vi "PS-RA01B FPGA Testbench.vi"() -> ()   [LabVIEW 2011]
uses:
  <vilib>/rvi/eio/common/nirviEmuTemplateMethod_errors.vi
  <vilib>/rvi/Memory/Memory_Emulation/niFpgaMemoryEmulationValidateCache.vi
  <vilib>/rvi/DataTransferAndStorage/Container/Common/niFpgaContainerGetUniqueNameForEmu.vi
  <vilib>/rvi/Memory/Memory_Emulation/nirvimemoryEmulationManagerCache_InsertValue.vi
  <vilib>/Utility/error.llb/Clear Errors.vi
  <vilib>/rvi/Memory/Memory_Emulation/nirvimemoryEmulationManagerCache_GetValue.vi
  <vilib>/rvi/Memory/Memory_Emulation/nirvimemoryEmulationManagerCache_SetValue.vi
  <vilib>/eio/EIONode/EIONode.xnode
  <vilib>/eio/EIOMethodNode/EIOMethodNode.xnode
  <vilib>/rvi/DataTransferAndStorage/Container/XNode/niFpgaContainer.xnode
  <vilib>/rvi/Memory/Memory_Emulation/nirvimemoryEmulation.vi
panel:
  out "ADDR":u8
  out "Mod6/AO1":fxp<+/-,20,5> format="%.17g"
  out "Mod2/AO3":fxp<+/-,20,5> format="%.17g"
  out "Mod2/AO2":fxp<+/-,20,5> format="%.17g"
  out "Mod2/AO1":fxp<+/-,20,5> format="%.17g"
  out "Mod2/AO0":fxp<+/-,20,5> format="%.17g"
  out "Mod6/AO3":fxp<+/-,20,5> format="%.17g"
  out "Mod6/AO2":fxp<+/-,20,5> format="%.17g"
  out "Mod6/AO0":fxp<+/-,20,5> format="%.17g"
  out "Timestamp":u32 caption="Tick Count(Ticks)"
  out "Mod5/AI0":fxp<+/-,20,5> format="%.17g"
  out "Mod5/AI2":fxp<+/-,20,5> format="%.17g"
  out "Mod5/AI3":fxp<+/-,20,5> format="%.17g"
  out "Mod1/AI0":fxp<+/-,20,5> format="%.17g"
  out "Mod1/AI1":fxp<+/-,20,5> format="%.17g"
  out "Mod1/AI2":fxp<+/-,20,5> format="%.17g"
  out "Mod1/AI3":fxp<+/-,20,5> format="%.17g"
  out "Mod5/AI1":fxp<+/-,20,5> format="%.17g"
  out "period":u32
  out "delay":u32
  out "dperiod":u32
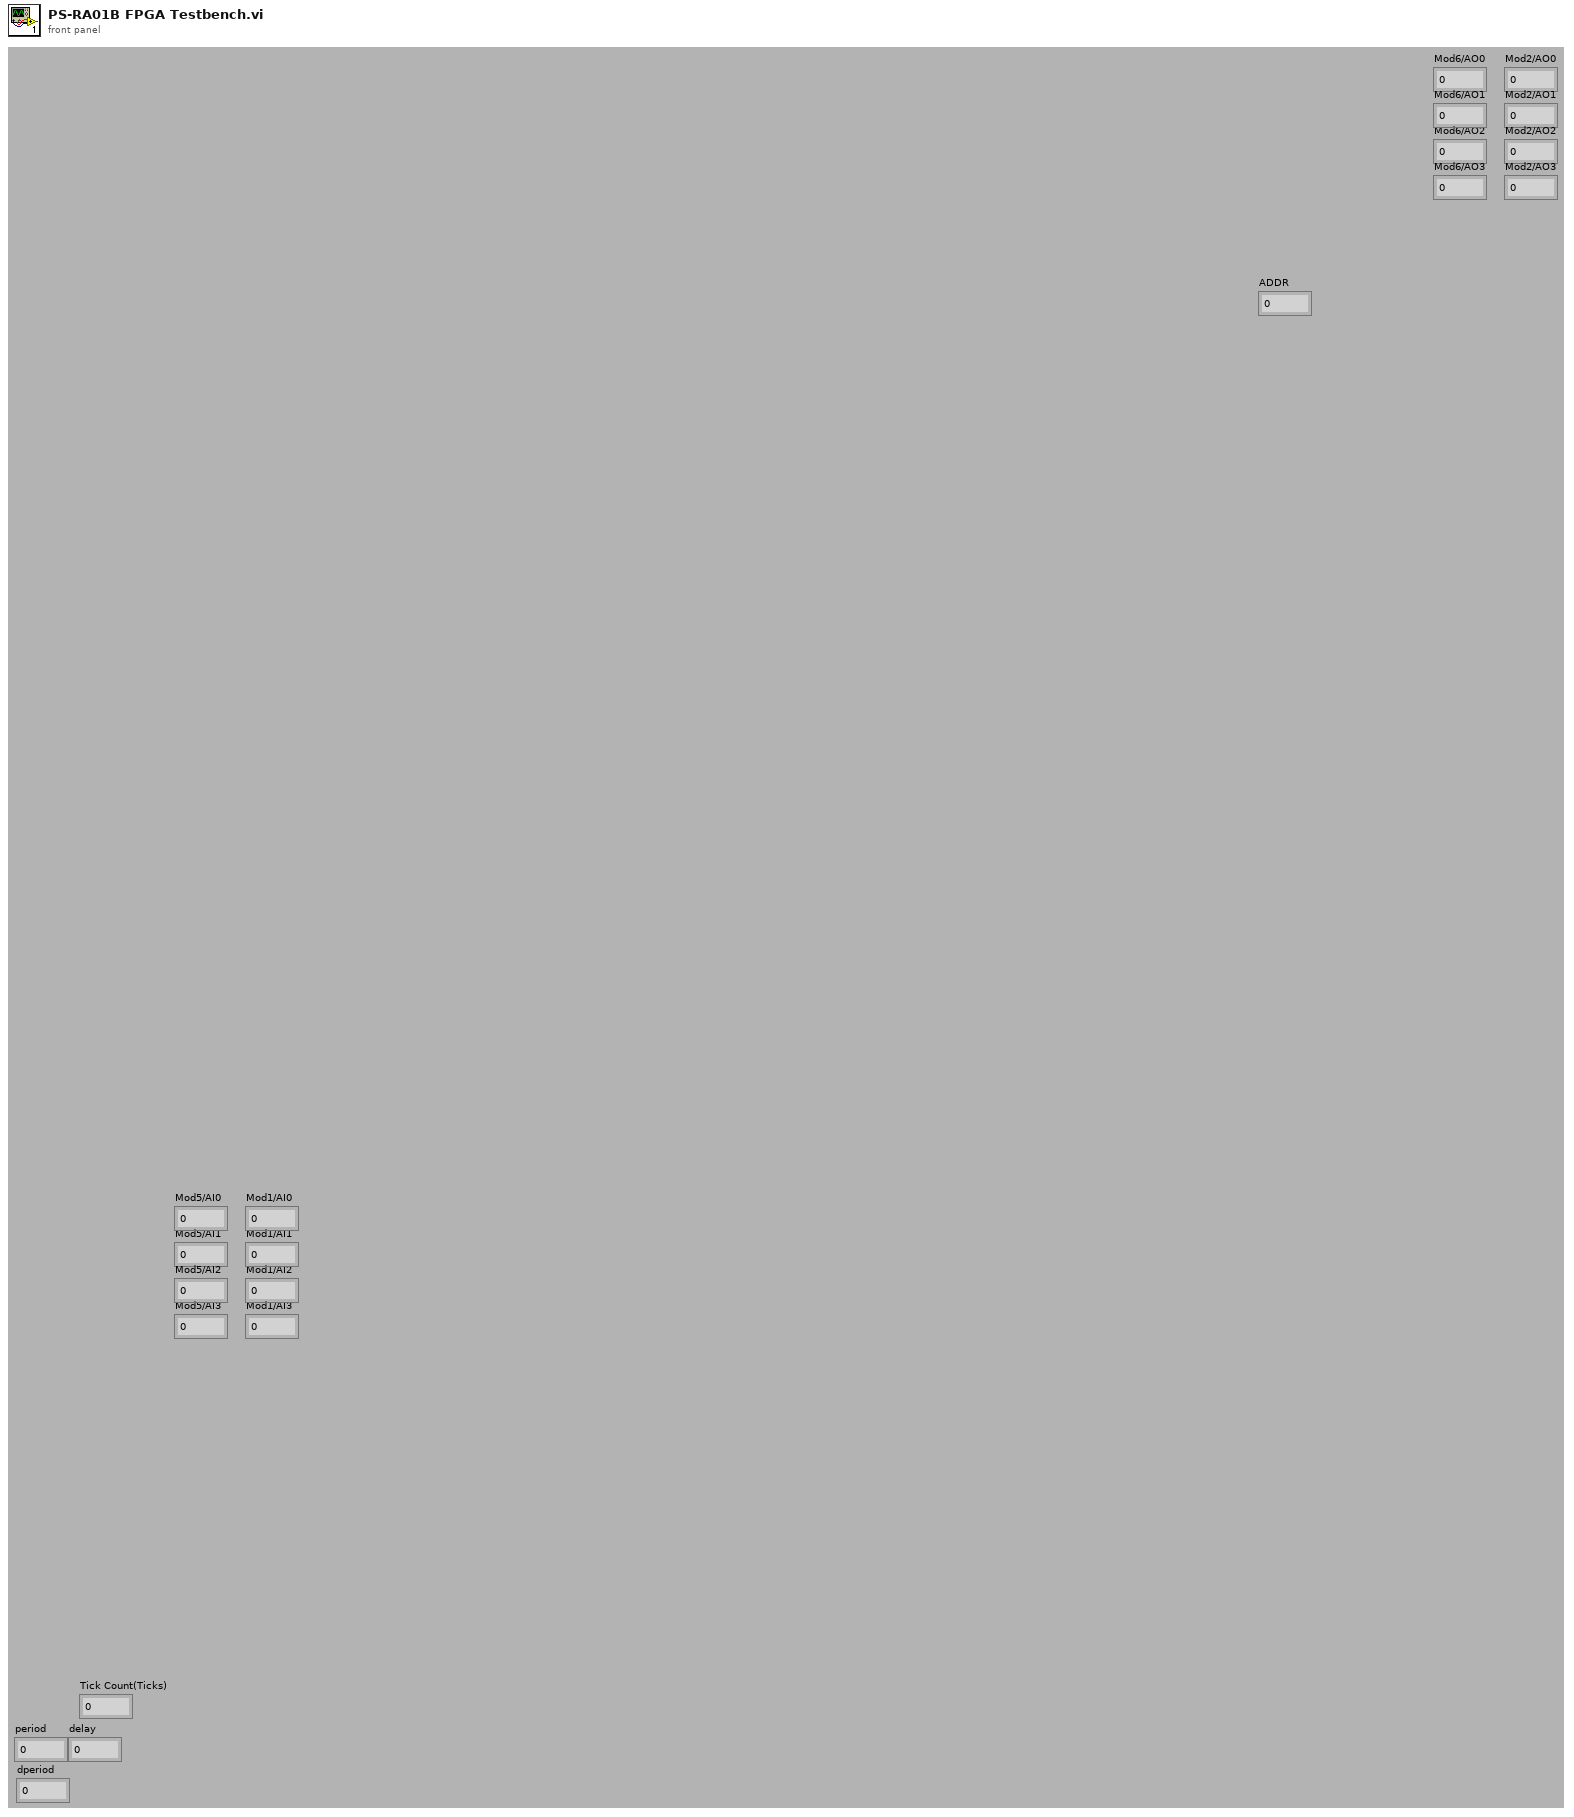
[diagram p1: front panel]
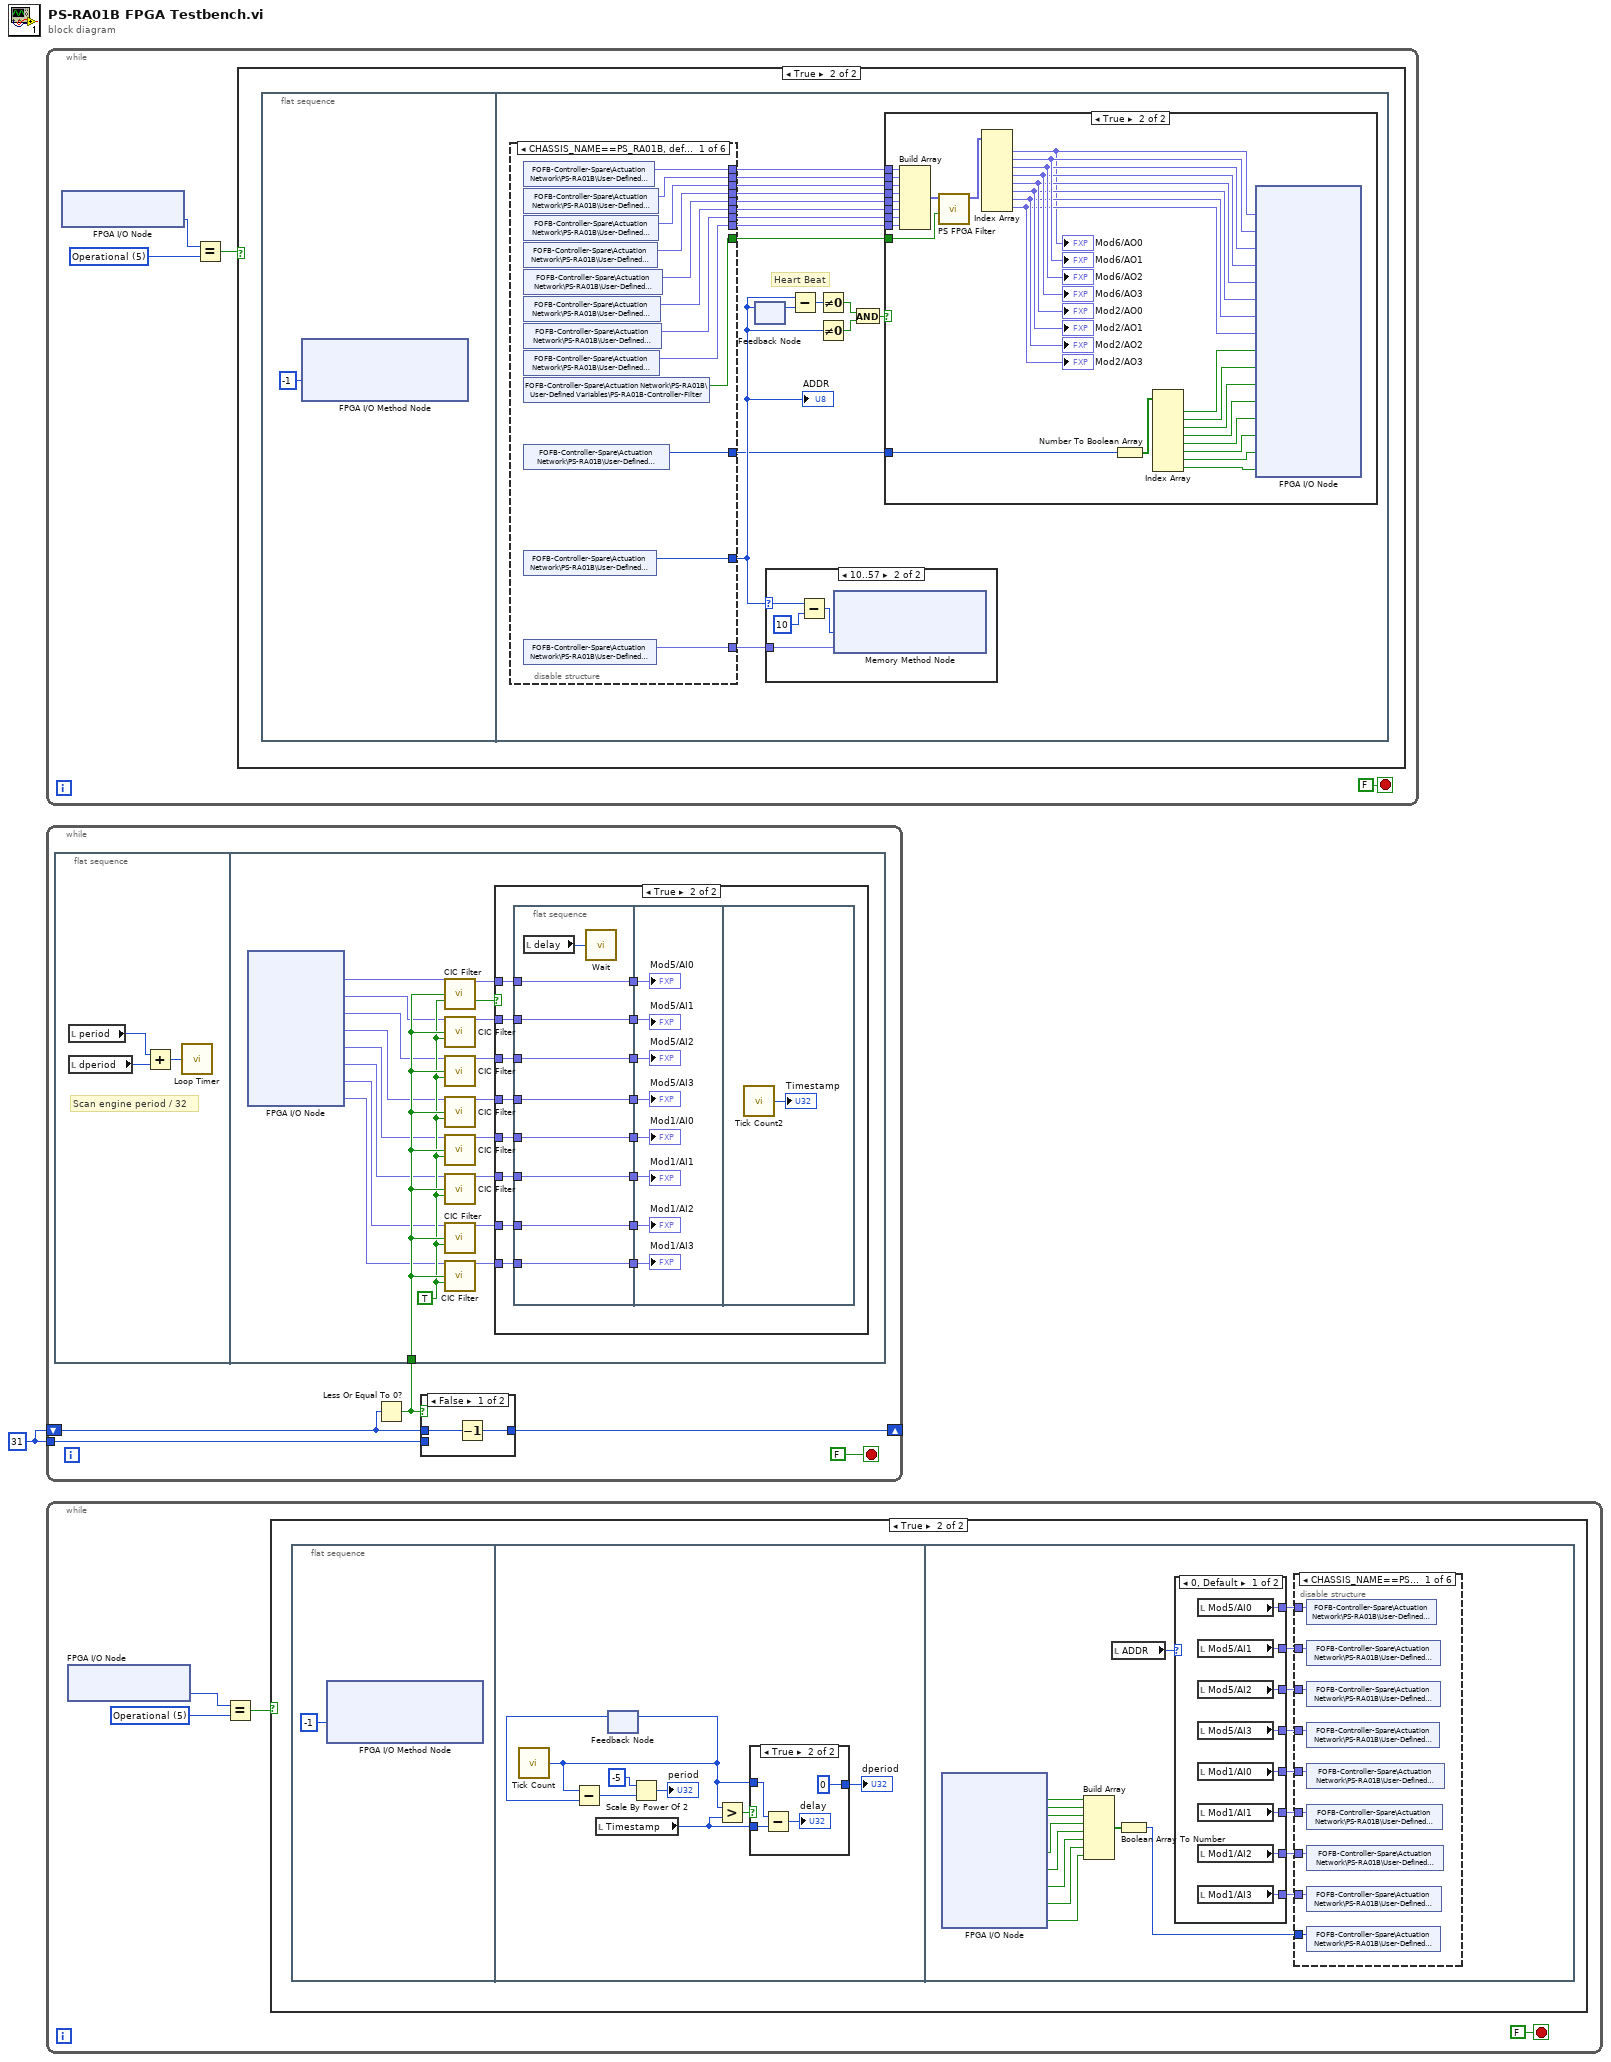
[diagram p0: block diagram]
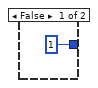
[diagram p5: hidden frame]
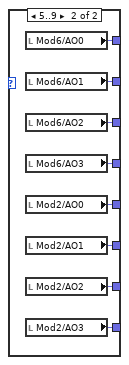
[diagram p6: hidden frame]
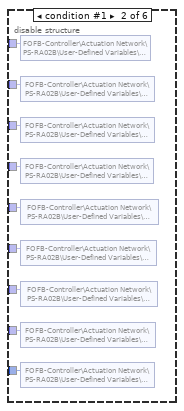
[diagram p7: hidden frame]
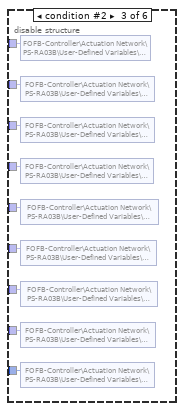
[diagram p8: hidden frame]
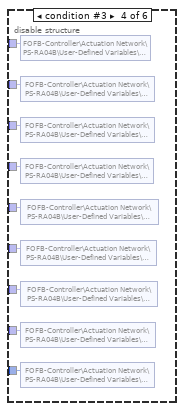
[diagram p9: hidden frame]
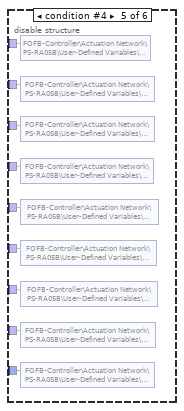
[diagram p10: hidden frame]
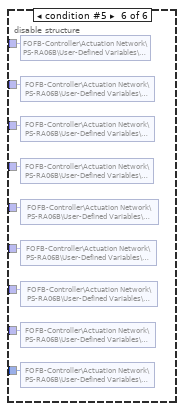
[diagram p11: hidden frame]
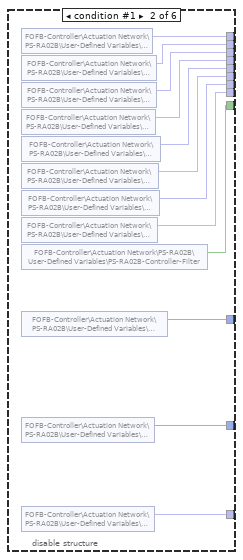
[diagram p15: hidden frame]
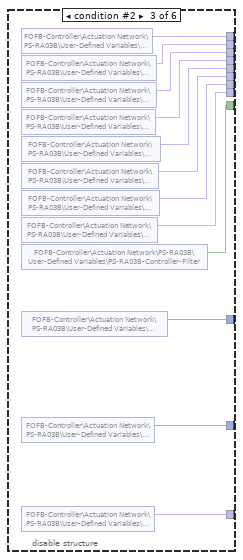
[diagram p16: hidden frame]
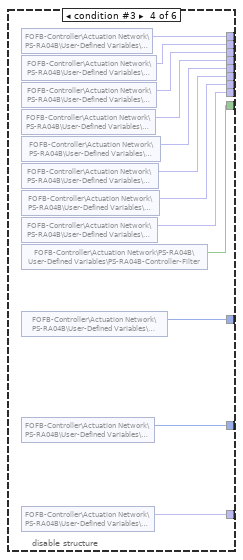
[diagram p17: hidden frame]
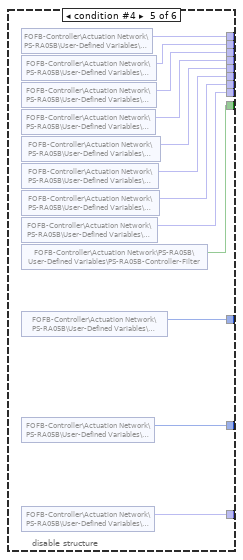
[diagram p18: hidden frame]
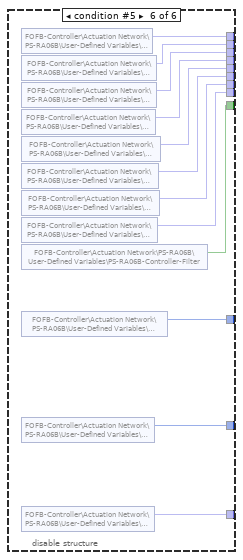
[diagram p19: hidden frame]
diagram:
  w1 = 31
  n1 = while {
    stop <- FALSE stop-if-true
    w2 = u8 5 items=["Init"=1, "PreOp"=2, "Bootstrap"=3, "SafeOp"=4, "Operational"=5]
    n2 = xnode "FPGA I/O Node"() -> ("EtherCAT State"=w3:u8)  [unwired: 1 in, 1 out]
    n3 = Equal?(x=w3, y=w2) -> (x = y?=w4:bool)
    n4 = case shown="True" w4 {
      frame False {
      }
      frame True {
        n5 = flat-sequence {
          frame #0 {
            n6 = xnode "FPGA I/O Method Node"("Timeout"=-1) -> ()  [unwired: 1 in, 2 out]
          }
          frame #1 {
            # "Heart Beat"
            n7 = disable-structure shown="CHASSIS_NAME==PS_RA01B, default" {
              disable-tunnel: [w68 w69 w82 w100 w112 w128] -> w23
              disable-tunnel: [w67 w70 w83 w99 w111 w123] -> w22
              disable-tunnel: [w66 w71 w84 w98 w110 w122] -> w21
              disable-tunnel: [w65 w72 w85 w97 w109 w121] -> w20
              disable-tunnel: [w64 w73 w86 w96 w108 w120] -> w19
              disable-tunnel: [w63 w74 w87 w95 w107 w119] -> w18
              disable-tunnel: [w62 w75 w88 w94 w106 w118] -> w17
              disable-tunnel: [w61 w76 w89 w93 w105 w117] -> w16
              disable-tunnel: [w60 w80 w92 w104 w116 w127] -> w7
              disable-tunnel: [w59 w79 w91 w103 w115 w126] -> w15
              disable-tunnel: [w58 w78 w90 w102 w114 w125] -> w13
              disable-tunnel: [w57 w77 w81 w101 w113 w124] -> w11
              frame condition #0 (active) {
                n8 = shared-variable "FOFB-Controller-Spare\\Actuation Network\\PS-RA01B\\User-Defined Variables\\ACH02-Setpoint"() -> (w68:fxp<+/-,20,5>)  [unwired: 1 in, 1 out]
                n9 = shared-variable "FOFB-Controller-Spare\\Actuation Network\\PS-RA01B\\User-Defined Variables\\RRA01B-Setpoint"() -> (w67:fxp<+/-,20,5>)  [unwired: 1 in, 1 out]
                n10 = shared-variable "FOFB-Controller-Spare\\Actuation Network\\PS-RA01B\\User-Defined Variables\\ALV02A-Setpoint"() -> (w66:fxp<+/-,20,5>)  [unwired: 1 in, 1 out]
                n11 = shared-variable "FOFB-Controller-Spare\\Actuation Network\\PS-RA01B\\User-Defined Variables\\ALV02B-Setpoint"() -> (w65:fxp<+/-,20,5>)  [unwired: 1 in, 1 out]
                n12 = shared-variable "FOFB-Controller-Spare\\Actuation Network\\PS-RA01B\\User-Defined Variables\\ACH03A-Setpoint"() -> (w64:fxp<+/-,20,5>)  [unwired: 1 in, 1 out]
                n13 = shared-variable "FOFB-Controller-Spare\\Actuation Network\\PS-RA01B\\User-Defined Variables\\ACV03A-Setpoint"() -> (w63:fxp<+/-,20,5>)  [unwired: 1 in, 1 out]
                n14 = shared-variable "FOFB-Controller-Spare\\Actuation Network\\PS-RA01B\\User-Defined Variables\\ACH01B-Setpoint"() -> (w62:fxp<+/-,20,5>)  [unwired: 1 in, 1 out]
                n15 = shared-variable "FOFB-Controller-Spare\\Actuation Network\\PS-RA01B\\User-Defined Variables\\ACV01B-Setpoint"() -> (w61:fxp<+/-,20,5>)  [unwired: 1 in, 1 out]
                n16 = shared-variable "FOFB-Controller-Spare\\Actuation Network\\PS-RA01B\\User-Defined Variables\\PS-RA01B-Controller-Filter"() -> (w59:bool)  [unwired: 1 in, 1 out]
                n17 = shared-variable "FOFB-Controller-Spare\\Actuation Network\\PS-RA01B\\User-Defined Variables\\PS-RA01B-ON-OFF"() -> (w60:u8)  [unwired: 1 in, 1 out]
                n18 = shared-variable "FOFB-Controller-Spare\\Actuation Network\\PS-RA01B\\User-Defined Variables\\PS-RA01B-ADDR"() -> (w57:u8)  [unwired: 1 in, 1 out]
                n19 = shared-variable "FOFB-Controller-Spare\\Actuation Network\\PS-RA01B\\User-Defined Variables\\PS-RA01B-DATA"() -> (w58:fxp<+/-,20,2>)  [unwired: 1 in, 1 out]
              }
              frame condition #1 {
                n20 = shared-variable "FOFB-Controller\\Actuation Network\\PS-RA02B\\User-Defined Variables\\ACH04-Setpoint"() -> (w69:fxp<+/-,20,5>)  [unwired: 1 in, 1 out]
                n21 = shared-variable "FOFB-Controller\\Actuation Network\\PS-RA02B\\User-Defined Variables\\RRA02B-Setpoint"() -> (w70:fxp<+/-,20,5>)  [unwired: 1 in, 1 out]
                n22 = shared-variable "FOFB-Controller\\Actuation Network\\PS-RA02B\\User-Defined Variables\\ALV04A-Setpoint"() -> (w71:fxp<+/-,20,5>)  [unwired: 1 in, 1 out]
                n23 = shared-variable "FOFB-Controller\\Actuation Network\\PS-RA02B\\User-Defined Variables\\ALV04B-Setpoint"() -> (w72:fxp<+/-,20,5>)  [unwired: 1 in, 1 out]
                n24 = shared-variable "FOFB-Controller\\Actuation Network\\PS-RA02B\\User-Defined Variables\\ACH05A-Setpoint"() -> (w73:fxp<+/-,20,5>)  [unwired: 1 in, 1 out]
                n25 = shared-variable "FOFB-Controller\\Actuation Network\\PS-RA02B\\User-Defined Variables\\ACV05A-Setpoint"() -> (w74:fxp<+/-,20,5>)  [unwired: 1 in, 1 out]
                n26 = shared-variable "FOFB-Controller\\Actuation Network\\PS-RA02B\\User-Defined Variables\\ACH03B-Setpoint"() -> (w75:fxp<+/-,20,5>)  [unwired: 1 in, 1 out]
                n27 = shared-variable "FOFB-Controller\\Actuation Network\\PS-RA02B\\User-Defined Variables\\ACV03B-Setpoint"() -> (w76:fxp<+/-,20,5>)  [unwired: 1 in, 1 out]
                n28 = shared-variable "FOFB-Controller\\Actuation Network\\PS-RA02B\\User-Defined Variables\\PS-RA02B-Controller-Filter"() -> (w79:bool)  [unwired: 1 in, 1 out]
                n29 = shared-variable "FOFB-Controller\\Actuation Network\\PS-RA02B\\User-Defined Variables\\PS-RA02B-ON-OFF"() -> (w80:u8)  [unwired: 1 in, 1 out]
                n30 = shared-variable "FOFB-Controller\\Actuation Network\\PS-RA02B\\User-Defined Variables\\PS-RA02B-ADDR"() -> (w77:u8)  [unwired: 1 in, 1 out]
                n31 = shared-variable "FOFB-Controller\\Actuation Network\\PS-RA02B\\User-Defined Variables\\PS-RA02B-DATA"() -> (w78:fxp<+/-,20,2>)  [unwired: 1 in, 1 out]
              }
              frame condition #2 {
                n32 = shared-variable "FOFB-Controller\\Actuation Network\\PS-RA03B\\User-Defined Variables\\ACH06-Setpoint"() -> (w82:fxp<+/-,20,5>)  [unwired: 1 in, 1 out]
                n33 = shared-variable "FOFB-Controller\\Actuation Network\\PS-RA03B\\User-Defined Variables\\RRA03B-Setpoint"() -> (w83:fxp<+/-,20,5>)  [unwired: 1 in, 1 out]
                n34 = shared-variable "FOFB-Controller\\Actuation Network\\PS-RA03B\\User-Defined Variables\\ALV06A-Setpoint"() -> (w84:fxp<+/-,20,5>)  [unwired: 1 in, 1 out]
                n35 = shared-variable "FOFB-Controller\\Actuation Network\\PS-RA03B\\User-Defined Variables\\ALV06B-Setpoint"() -> (w85:fxp<+/-,20,5>)  [unwired: 1 in, 1 out]
                n36 = shared-variable "FOFB-Controller\\Actuation Network\\PS-RA03B\\User-Defined Variables\\ACH07A-Setpoint"() -> (w86:fxp<+/-,20,5>)  [unwired: 1 in, 1 out]
                n37 = shared-variable "FOFB-Controller\\Actuation Network\\PS-RA03B\\User-Defined Variables\\ACV07A-Setpoint"() -> (w87:fxp<+/-,20,5>)  [unwired: 1 in, 1 out]
                n38 = shared-variable "FOFB-Controller\\Actuation Network\\PS-RA03B\\User-Defined Variables\\ACH05B-Setpoint"() -> (w88:fxp<+/-,20,5>)  [unwired: 1 in, 1 out]
                n39 = shared-variable "FOFB-Controller\\Actuation Network\\PS-RA03B\\User-Defined Variables\\ACV05B-Setpoint"() -> (w89:fxp<+/-,20,5>)  [unwired: 1 in, 1 out]
                n40 = shared-variable "FOFB-Controller\\Actuation Network\\PS-RA03B\\User-Defined Variables\\PS-RA03B-Controller-Filter"() -> (w91:bool)  [unwired: 1 in, 1 out]
                n41 = shared-variable "FOFB-Controller\\Actuation Network\\PS-RA03B\\User-Defined Variables\\PS-RA03B-ON-OFF"() -> (w92:u8)  [unwired: 1 in, 1 out]
                n42 = shared-variable "FOFB-Controller\\Actuation Network\\PS-RA03B\\User-Defined Variables\\PS-RA03B-ADDR"() -> (w81:u8)  [unwired: 1 in, 1 out]
                n43 = shared-variable "FOFB-Controller\\Actuation Network\\PS-RA03B\\User-Defined Variables\\PS-RA03B-DATA"() -> (w90:fxp<+/-,20,2>)  [unwired: 1 in, 1 out]
              }
              frame condition #3 {
                n44 = shared-variable "FOFB-Controller\\Actuation Network\\PS-RA04B\\User-Defined Variables\\ACH08-Setpoint"() -> (w100:fxp<+/-,20,5>)  [unwired: 1 in, 1 out]
                n45 = shared-variable "FOFB-Controller\\Actuation Network\\PS-RA04B\\User-Defined Variables\\RRA04B-Setpoint"() -> (w99:fxp<+/-,20,5>)  [unwired: 1 in, 1 out]
                n46 = shared-variable "FOFB-Controller\\Actuation Network\\PS-RA04B\\User-Defined Variables\\ALV08A-Setpoint"() -> (w98:fxp<+/-,20,5>)  [unwired: 1 in, 1 out]
                n47 = shared-variable "FOFB-Controller\\Actuation Network\\PS-RA04B\\User-Defined Variables\\ALV08B-Setpoint"() -> (w97:fxp<+/-,20,5>)  [unwired: 1 in, 1 out]
                n48 = shared-variable "FOFB-Controller\\Actuation Network\\PS-RA04B\\User-Defined Variables\\ACH09A-Setpoint"() -> (w96:fxp<+/-,20,5>)  [unwired: 1 in, 1 out]
                n49 = shared-variable "FOFB-Controller\\Actuation Network\\PS-RA04B\\User-Defined Variables\\ACV09A-Setpoint"() -> (w95:fxp<+/-,20,5>)  [unwired: 1 in, 1 out]
                n50 = shared-variable "FOFB-Controller\\Actuation Network\\PS-RA04B\\User-Defined Variables\\ACH07B-Setpoint"() -> (w94:fxp<+/-,20,5>)  [unwired: 1 in, 1 out]
                n51 = shared-variable "FOFB-Controller\\Actuation Network\\PS-RA04B\\User-Defined Variables\\ACV07B-Setpoint"() -> (w93:fxp<+/-,20,5>)  [unwired: 1 in, 1 out]
                n52 = shared-variable "FOFB-Controller\\Actuation Network\\PS-RA04B\\User-Defined Variables\\PS-RA04B-Controller-Filter"() -> (w103:bool)  [unwired: 1 in, 1 out]
                n53 = shared-variable "FOFB-Controller\\Actuation Network\\PS-RA04B\\User-Defined Variables\\PS-RA04B-ON-OFF"() -> (w104:u8)  [unwired: 1 in, 1 out]
                n54 = shared-variable "FOFB-Controller\\Actuation Network\\PS-RA04B\\User-Defined Variables\\PS-RA04B-ADDR"() -> (w101:u8)  [unwired: 1 in, 1 out]
                n55 = shared-variable "FOFB-Controller\\Actuation Network\\PS-RA04B\\User-Defined Variables\\PS-RA04B-DATA"() -> (w102:fxp<+/-,20,2>)  [unwired: 1 in, 1 out]
              }
              frame condition #4 {
                n56 = shared-variable "FOFB-Controller\\Actuation Network\\PS-RA05B\\User-Defined Variables\\ACH10-Setpoint"() -> (w112:fxp<+/-,20,5>)  [unwired: 1 in, 1 out]
                n57 = shared-variable "FOFB-Controller\\Actuation Network\\PS-RA05B\\User-Defined Variables\\RRA05B-Setpoint"() -> (w111:fxp<+/-,20,5>)  [unwired: 1 in, 1 out]
                n58 = shared-variable "FOFB-Controller\\Actuation Network\\PS-RA05B\\User-Defined Variables\\ALV10A-Setpoint"() -> (w110:fxp<+/-,20,5>)  [unwired: 1 in, 1 out]
                n59 = shared-variable "FOFB-Controller\\Actuation Network\\PS-RA05B\\User-Defined Variables\\ALV10B-Setpoint"() -> (w109:fxp<+/-,20,5>)  [unwired: 1 in, 1 out]
                n60 = shared-variable "FOFB-Controller\\Actuation Network\\PS-RA05B\\User-Defined Variables\\ACH11A-Setpoint"() -> (w108:fxp<+/-,20,5>)  [unwired: 1 in, 1 out]
                n61 = shared-variable "FOFB-Controller\\Actuation Network\\PS-RA05B\\User-Defined Variables\\ACV11A-Setpoint"() -> (w107:fxp<+/-,20,5>)  [unwired: 1 in, 1 out]
                n62 = shared-variable "FOFB-Controller\\Actuation Network\\PS-RA05B\\User-Defined Variables\\ACH09B-Setpoint"() -> (w106:fxp<+/-,20,5>)  [unwired: 1 in, 1 out]
                n63 = shared-variable "FOFB-Controller\\Actuation Network\\PS-RA05B\\User-Defined Variables\\ACV09B-Setpoint"() -> (w105:fxp<+/-,20,5>)  [unwired: 1 in, 1 out]
                n64 = shared-variable "FOFB-Controller\\Actuation Network\\PS-RA05B\\User-Defined Variables\\PS-RA05B-Controller-Filter"() -> (w115:bool)  [unwired: 1 in, 1 out]
                n65 = shared-variable "FOFB-Controller\\Actuation Network\\PS-RA05B\\User-Defined Variables\\PS-RA05B-ON-OFF"() -> (w116:u8)  [unwired: 1 in, 1 out]
                n66 = shared-variable "FOFB-Controller\\Actuation Network\\PS-RA05B\\User-Defined Variables\\PS-RA05B-ADDR"() -> (w113:u8)  [unwired: 1 in, 1 out]
                n67 = shared-variable "FOFB-Controller\\Actuation Network\\PS-RA05B\\User-Defined Variables\\PS-RA05B-DATA"() -> (w114:fxp<+/-,20,2>)  [unwired: 1 in, 1 out]
              }
              frame condition #5 {
                n68 = shared-variable "FOFB-Controller\\Actuation Network\\PS-RA06B\\User-Defined Variables\\ACH12-Setpoint"() -> (w128:fxp<+/-,20,5>)  [unwired: 1 in, 1 out]
                n69 = shared-variable "FOFB-Controller\\Actuation Network\\PS-RA06B\\User-Defined Variables\\RRA06B-Setpoint"() -> (w123:fxp<+/-,20,5>)  [unwired: 1 in, 1 out]
                n70 = shared-variable "FOFB-Controller\\Actuation Network\\PS-RA06B\\User-Defined Variables\\ALV12A-Setpoint"() -> (w122:fxp<+/-,20,5>)  [unwired: 1 in, 1 out]
                n71 = shared-variable "FOFB-Controller\\Actuation Network\\PS-RA06B\\User-Defined Variables\\ALV12B-Setpoint"() -> (w121:fxp<+/-,20,5>)  [unwired: 1 in, 1 out]
                n72 = shared-variable "FOFB-Controller\\Actuation Network\\PS-RA06B\\User-Defined Variables\\ACH01A-Setpoint"() -> (w120:fxp<+/-,20,5>)  [unwired: 1 in, 1 out]
                n73 = shared-variable "FOFB-Controller\\Actuation Network\\PS-RA06B\\User-Defined Variables\\ACV01A-Setpoint"() -> (w119:fxp<+/-,20,5>)  [unwired: 1 in, 1 out]
                n74 = shared-variable "FOFB-Controller\\Actuation Network\\PS-RA06B\\User-Defined Variables\\ACH11B-Setpoint"() -> (w118:fxp<+/-,20,5>)  [unwired: 1 in, 1 out]
                n75 = shared-variable "FOFB-Controller\\Actuation Network\\PS-RA06B\\User-Defined Variables\\ACV11B-Setpoint"() -> (w117:fxp<+/-,20,5>)  [unwired: 1 in, 1 out]
                n76 = shared-variable "FOFB-Controller\\Actuation Network\\PS-RA06B\\User-Defined Variables\\PS-RA06B-Controller-Filter"() -> (w126:bool)  [unwired: 1 in, 1 out]
                n77 = shared-variable "FOFB-Controller\\Actuation Network\\PS-RA06B\\User-Defined Variables\\PS-RA06B-ON-OFF"() -> (w127:u8)  [unwired: 1 in, 1 out]
                n78 = shared-variable "FOFB-Controller\\Actuation Network\\PS-RA06B\\User-Defined Variables\\PS-RA06B-ADDR"() -> (w124:u8)  [unwired: 1 in, 1 out]
                n79 = shared-variable "FOFB-Controller\\Actuation Network\\PS-RA06B\\User-Defined Variables\\PS-RA06B-DATA"() -> (w125:fxp<+/-,20,2>)  [unwired: 1 in, 1 out]
              }
            }
            "ADDR" <- w11
            n80 = feedback #1() -> (w14:u8)  [unwired: 1 in]
            n81 = feedback-in #1(w11) -> ()
            n82 = case shown="10..57" w11 {
              selector: w11 -> [_ w27]
              tunnel: w13 -> [_ w24]
              frame 0, Default {
              }
              frame 10..57 {
                n83 = Subtract(x=w27, y=u8 10) -> (x-y=w25:u8)
                n84 = xnode ("Memory Method Node")("Address"=w25, "Data"=w24) -> ()  [unwired: 1 in, 1 out]
              }
            }
            n85 = Subtract(x=w11, y=w14) -> (x-y=w12:i8)
            n86 = Not Equal To 0?(x=w12) -> (x != 0?=w10:bool)
            n87 = Not Equal To 0?(x=w11) -> (x != 0?=w9:bool)
            n88 = And(x=w10, y=w9) -> (x .and. y?=w8:bool)
            n89 = case shown="True" w8 {
              tunnel: w23 -> [_ w56]
              tunnel: w22 -> [_ w55]
              tunnel: w21 -> [_ w54]
              tunnel: w20 -> [_ w53]
              tunnel: w19 -> [_ w52]
              tunnel: w18 -> [_ w51]
              tunnel: w17 -> [_ w50]
              tunnel: w16 -> [_ w49]
              tunnel: w15 -> [_ w46]
              tunnel: w7 -> [_ w37]
              frame False {
              }
              frame True {
                n90 = Build Array(w56, w55, w54, w53, w52, w51, w50, w49) -> (w48:fxp<+/-,20,5>[])
                n91 = call "PS FPGA Filter.vi"("loop?"=w46, "input"=w48) -> ("output"=w47:fxp<+/-,20,5>[])  [unwired: 9 in]
                n92 = Index Array(array=w47) -> (element #1=w28:fxp<+/-,20,5>, element #2=w45:fxp<+/-,20,5>, element #3=w44:fxp<+/-,20,5>, element #4=w43:fxp<+/-,20,5>, element #5=w42:fxp<+/-,20,5>, element #6=w41:fxp<+/-,20,5>, element #7=w40:fxp<+/-,20,5>, element #8=w39:fxp<+/-,20,5>)  [unwired: 8 in]
                "Mod6/AO0" <- w28
                "Mod6/AO2" <- w44
                "Mod6/AO3" <- w43
                "Mod2/AO0" <- w42
                "Mod2/AO1" <- w41
                "Mod2/AO2" <- w40
                "Mod2/AO3" <- w39
                "Mod6/AO1" <- w45
                n93 = Number To Boolean Array(number=w37) -> (Boolean array=w38:bool[])
                n94 = Index Array(array=w38) -> (element #1=w36:bool, element #2=w35:bool, element #3=w34:bool, element #4=w33:bool, element #5=w32:bool, element #6=w29:bool, element #7=w30:bool, element #8=w31:bool)  [unwired: 8 in]
                n95 = xnode "FPGA I/O Node"("Mod6/AO0"=w28, "Mod6/AO1"=w45, "Mod6/AO2"=w44, "Mod6/AO3"=w43, "Mod2/AO0"=w42, "Mod2/AO1"=w41, "Mod2/AO2"=w40, "Mod2/AO3"=w39, "Mod4/DIO6"=w36, "Mod4/DIO7"=w35, "Mod4/DIO4"=w34, "Mod4/DIO5"=w33, "Mod4/DIO2"=w32, "Mod4/DIO3"=w29, "Mod4/DIO0"=w30, "Mod4/DIO1"=w31) -> ()  [unwired: 16 in, 16 out]
              }
            }
          }
        }
      }
    }
  }
  n96 = while {
    shift-right: [w132] -> _
    shift-left: w1 -> [w131]
    tunnel: w1 -> [w129]
    stop <- FALSE stop-if-true
    n97 = flat-sequence {
      tunnel: w130 -> [w158]
      frame #0 {
        # "Scan engine period / 32"
        n98 = local read "period"() -> (w139:u32)
        n99 = local read "dperiod"() -> (w138:u32)
        n100 = Add(x=w139, y=w138) -> (x+y=w137:u32)
        n101 = call "Loop Timer"("Count(Ticks)"=w137) -> ()  [unwired: 1 out]
      }
      frame #1 {
        w157 = TRUE ("input valid")
        n102 = xnode "FPGA I/O Node"() -> ("Mod5/AI0"=w156:fxp<+/-,20,5>, "Mod5/AI1"=w155:fxp<+/-,20,5>, "Mod5/AI2"=w154:fxp<+/-,20,5>, "Mod5/AI3"=w153:fxp<+/-,20,5>, "Mod1/AI0"=w152:fxp<+/-,20,5>, "Mod1/AI1"=w151:fxp<+/-,20,5>, "Mod1/AI2"=w150:fxp<+/-,20,5>, "Mod1/AI3"=w149:fxp<+/-,20,5>)  [unwired: 8 in, 8 out]
        n103 = call "CIC Filter.vi"("input data"=w156, "sample"=w158, "input valid"=w157) -> ("output data"=w147:fxp<+/-,20,5>, "output valid"=w148:bool)  [unwired: 10 in, 1 out]
        n104 = call "CIC Filter.vi"("input data"=w155, "sample"=w158, "input valid"=w157) -> ("output data"=w146:fxp<+/-,20,5>)  [unwired: 10 in, 2 out]
        n105 = call "CIC Filter.vi"("input data"=w154, "sample"=w158, "input valid"=w157) -> ("output data"=w145:fxp<+/-,20,5>)  [unwired: 10 in, 2 out]
        n106 = call "CIC Filter.vi"("input data"=w153, "sample"=w158, "input valid"=w157) -> ("output data"=w144:fxp<+/-,20,5>)  [unwired: 10 in, 2 out]
        n107 = call "CIC Filter.vi"("input data"=w152, "sample"=w158, "input valid"=w157) -> ("output data"=w143:fxp<+/-,20,5>)  [unwired: 10 in, 2 out]
        n108 = call "CIC Filter.vi"("input data"=w151, "sample"=w158, "input valid"=w157) -> ("output data"=w142:fxp<+/-,20,5>)  [unwired: 10 in, 2 out]
        n109 = call "CIC Filter.vi"("input data"=w150, "sample"=w158, "input valid"=w157) -> ("output data"=w141:fxp<+/-,20,5>)  [unwired: 10 in, 2 out]
        n110 = call "CIC Filter.vi"("input data"=w149, "sample"=w158, "input valid"=w157) -> ("output data"=w140:fxp<+/-,20,5>)  [unwired: 10 in, 2 out]
        n111 = case shown="True" w148 {
          tunnel: w147 -> [_ w174]
          tunnel: w146 -> [_ w172]
          tunnel: w145 -> [_ w170]
          tunnel: w144 -> [_ w169]
          tunnel: w143 -> [_ w166]
          tunnel: w142 -> [_ w164]
          tunnel: w141 -> [_ w162]
          tunnel: w140 -> [_ w160]
          frame False {
          }
          frame True {
            n112 = flat-sequence {
              tunnel: w174 -> [w183]
              tunnel: [w183] -> w173
              tunnel: w172 -> [w181]
              tunnel: [w181] -> w171
              tunnel: w170 -> [w179]
              tunnel: w169 -> [w180]
              tunnel: [w180] -> w168
              tunnel: [w179] -> w167
              tunnel: w166 -> [w178]
              tunnel: [w178] -> w165
              tunnel: w164 -> [w177]
              tunnel: [w177] -> w163
              tunnel: w162 -> [w176]
              tunnel: [w176] -> w161
              tunnel: w160 -> [w175]
              tunnel: [w175] -> w159
              tunnel: w173 -> [w190]
              tunnel: w171 -> [w191]
              tunnel: w168 -> [w189]
              tunnel: w167 -> [w188]
              tunnel: w165 -> [w187]
              tunnel: w163 -> [w186]
              tunnel: w161 -> [w185]
              tunnel: w159 -> [w184]
              frame #0 {
                n113 = local read "delay"() -> (w182:u32)
                n114 = call "Wait"("Count(Ticks)"=w182) -> ()  [unwired: 1 out]
              }
              frame #1 {
                "Mod5/AI0" <- w190
                "Mod5/AI2" <- w188
                "Mod5/AI3" <- w189
                "Mod1/AI0" <- w187
                "Mod1/AI1" <- w186
                "Mod1/AI2" <- w185
                "Mod1/AI3" <- w184
                "Mod5/AI1" <- w191
              }
              frame #2 {
                n115 = call "Tick Count2"() -> ("Tick Count(Ticks)"=→"Timestamp":u32)
              }
            }
          }
        }
      }
    }
    n116 = Less Or Equal To 0?(x=w131) -> (x <= 0?=w130:bool)
    n117 = case shown="False" w130 {
      tunnel: [w135 w136] -> w132
      tunnel: w131 -> [w134 _]
      tunnel: w129 -> [_ w136]
      frame False {
        n118 = Decrement(x=w134) -> (x-1=w135:i32)
      }
      frame True {
      }
    }
  }
  n119 = while {
    stop <- FALSE stop-if-true
    w195 = u8 5 items=["Init"=1, "PreOp"=2, "Bootstrap"=3, "SafeOp"=4, "Operational"=5]
    n120 = xnode "FPGA I/O Node"() -> ("EtherCAT State"=w194:u8)  [unwired: 1 in, 1 out]
    n121 = Equal?(x=w194, y=w195) -> (x = y?=w193:bool)
    n122 = case shown="True" w193 {
      frame False {
      }
      frame True {
        n123 = flat-sequence {
          frame #0 {
            n124 = xnode "FPGA I/O Method Node"("Timeout"=-1) -> ()  [unwired: 1 in, 2 out]
          }
          frame #1 {
            n125 = call "Tick Count"() -> ("Tick Count(Ticks)"=w199:u32)
            n126 = local read "Timestamp"() -> (w201:u32)
            n127 = feedback #2() -> (w198:u32)  [unwired: 1 in]
            n128 = Subtract(x=w199, y=w198) -> (x-y=w204:u32)
            n129 = feedback-in #2(w199) -> ()
            n130 = Scale By Power Of 2(n=i8 -5, x=w204) -> (x*2^n=→"period":u32)
            n131 = Greater?(x=w199, y=w201) -> (0:w202:bool)
            n132 = case shown="True" w202 {
              tunnel: w199 -> [_ w210]
              tunnel: w201 -> [_ w209]
              tunnel: [u32 1 ("dt 2") u32 0 ("dt 2")] -> w200
              frame False {
              }
              frame True {
                n133 = Subtract(x=w210, y=w209) -> (x-y=→"delay":u32)
              }
            }
            "dperiod" <- w200
          }
          frame #2 {
            n134 = xnode "FPGA I/O Node"() -> ("Mod3/DIO6"=w214:bool, "Mod3/DIO7"=w215:bool, "Mod3/DIO4"=w216:bool, "Mod3/DIO5"=w217:bool, "Mod3/DIO2"=w218:bool, "Mod3/DIO3"=w219:bool, "Mod3/DIO0"=w220:bool, "Mod3/DIO1"=w221:bool)  [unwired: 8 in, 8 out]
            n135 = Build Array(w214, w215, w216, w217, w218, w219, w220, w221) -> (w213:bool[])
            n136 = local read "ADDR"() -> (w211:u8)
            n137 = Boolean Array To Number(Boolean array=w213) -> (number=w212:u8)
            n138 = case shown="0, Default" w211 {
              tunnel: [w237 w245] -> w229
              tunnel: [w236 w244] -> w228
              tunnel: [w235 w243] -> w227
              tunnel: [w234 w238] -> w226
              tunnel: [w233 w239] -> w225
              tunnel: [w232 w240] -> w224
              tunnel: [w231 w241] -> w223
              tunnel: [w230 w242] -> w222
              frame 0, Default {
                n139 = local read "Mod5/AI0"() -> (w237:fxp<+/-,20,5>)
                n140 = local read "Mod5/AI1"() -> (w236:fxp<+/-,20,5>)
                n141 = local read "Mod5/AI2"() -> (w235:fxp<+/-,20,5>)
                n142 = local read "Mod5/AI3"() -> (w234:fxp<+/-,20,5>)
                n143 = local read "Mod1/AI0"() -> (w233:fxp<+/-,20,5>)
                n144 = local read "Mod1/AI1"() -> (w232:fxp<+/-,20,5>)
                n145 = local read "Mod1/AI2"() -> (w231:fxp<+/-,20,5>)
                n146 = local read "Mod1/AI3"() -> (w230:fxp<+/-,20,5>)
              }
              frame 5..9 {
                n147 = local read "Mod6/AO0"() -> (w245:fxp<+/-,20,5>)
                n148 = local read "Mod6/AO1"() -> (w244:fxp<+/-,20,5>)
                n149 = local read "Mod6/AO2"() -> (w243:fxp<+/-,20,5>)
                n150 = local read "Mod6/AO3"() -> (w238:fxp<+/-,20,5>)
                n151 = local read "Mod2/AO0"() -> (w239:fxp<+/-,20,5>)
                n152 = local read "Mod2/AO1"() -> (w240:fxp<+/-,20,5>)
                n153 = local read "Mod2/AO2"() -> (w241:fxp<+/-,20,5>)
                n154 = local read "Mod2/AO3"() -> (w242:fxp<+/-,20,5>)
              }
            }
            n155 = disable-structure shown="CHASSIS_NAME==PS_RA01B, default" {
              disable-tunnel: w229 -> [w254 w262 w271 w280 w289 w298]
              disable-tunnel: w228 -> [w253 w261 w270 w279 w288 w297]
              disable-tunnel: w227 -> [w252 w260 w269 w278 w287 w296]
              disable-tunnel: w226 -> [w251 w259 w268 w277 w286 w295]
              disable-tunnel: w225 -> [w250 w258 w267 w276 w285 w294]
              disable-tunnel: w224 -> [w249 w257 w266 w275 w284 w293]
              disable-tunnel: w223 -> [w248 w256 w265 w274 w283 w292]
              disable-tunnel: w222 -> [w247 w255 w264 w273 w282 w291]
              disable-tunnel: w212 -> [w246 w263 w272 w281 w290 w299]
              frame condition #0 (active) {
                n156 = shared-variable "FOFB-Controller-Spare\\Actuation Network\\PS-RA01B\\User-Defined Variables\\ACH02-Reading"(w254) -> ()  [unwired: 1 in, 1 out]
                n157 = shared-variable "FOFB-Controller-Spare\\Actuation Network\\PS-RA01B\\User-Defined Variables\\RRA01B-Reading"(w253) -> ()  [unwired: 1 in, 1 out]
                n158 = shared-variable "FOFB-Controller-Spare\\Actuation Network\\PS-RA01B\\User-Defined Variables\\ALV02A-Reading"(w252) -> ()  [unwired: 1 in, 1 out]
                n159 = shared-variable "FOFB-Controller-Spare\\Actuation Network\\PS-RA01B\\User-Defined Variables\\ALV02B-Reading"(w251) -> ()  [unwired: 1 in, 1 out]
                n160 = shared-variable "FOFB-Controller-Spare\\Actuation Network\\PS-RA01B\\User-Defined Variables\\ACH03A-Reading"(w250) -> ()  [unwired: 1 in, 1 out]
                n161 = shared-variable "FOFB-Controller-Spare\\Actuation Network\\PS-RA01B\\User-Defined Variables\\ACV03A-Reading"(w249) -> ()  [unwired: 1 in, 1 out]
                n162 = shared-variable "FOFB-Controller-Spare\\Actuation Network\\PS-RA01B\\User-Defined Variables\\ACH01B-Reading"(w248) -> ()  [unwired: 1 in, 1 out]
                n163 = shared-variable "FOFB-Controller-Spare\\Actuation Network\\PS-RA01B\\User-Defined Variables\\ACV01B-Reading"(w247) -> ()  [unwired: 1 in, 1 out]
                n164 = shared-variable "FOFB-Controller-Spare\\Actuation Network\\PS-RA01B\\User-Defined Variables\\PS-RA01B-Status"(w246) -> ()  [unwired: 1 in, 1 out]
              }
              frame condition #1 {
                n165 = shared-variable "FOFB-Controller\\Actuation Network\\PS-RA02B\\User-Defined Variables\\ACH04-Reading"(w262) -> ()  [unwired: 1 in, 1 out]
                n166 = shared-variable "FOFB-Controller\\Actuation Network\\PS-RA02B\\User-Defined Variables\\RRA02B-Reading"(w261) -> ()  [unwired: 1 in, 1 out]
                n167 = shared-variable "FOFB-Controller\\Actuation Network\\PS-RA02B\\User-Defined Variables\\ALV04A-Reading"(w260) -> ()  [unwired: 1 in, 1 out]
                n168 = shared-variable "FOFB-Controller\\Actuation Network\\PS-RA02B\\User-Defined Variables\\ALV04B-Reading"(w259) -> ()  [unwired: 1 in, 1 out]
                n169 = shared-variable "FOFB-Controller\\Actuation Network\\PS-RA02B\\User-Defined Variables\\ACH05A-Reading"(w258) -> ()  [unwired: 1 in, 1 out]
                n170 = shared-variable "FOFB-Controller\\Actuation Network\\PS-RA02B\\User-Defined Variables\\ACV05A-Reading"(w257) -> ()  [unwired: 1 in, 1 out]
                n171 = shared-variable "FOFB-Controller\\Actuation Network\\PS-RA02B\\User-Defined Variables\\ACH03B-Reading"(w256) -> ()  [unwired: 1 in, 1 out]
                n172 = shared-variable "FOFB-Controller\\Actuation Network\\PS-RA02B\\User-Defined Variables\\ACV03B-Reading"(w255) -> ()  [unwired: 1 in, 1 out]
                n173 = shared-variable "FOFB-Controller\\Actuation Network\\PS-RA02B\\User-Defined Variables\\PS-RA02B-Status"(w263) -> ()  [unwired: 1 in, 1 out]
              }
              frame condition #2 {
                n174 = shared-variable "FOFB-Controller\\Actuation Network\\PS-RA03B\\User-Defined Variables\\ACH06-Reading"(w271) -> ()  [unwired: 1 in, 1 out]
                n175 = shared-variable "FOFB-Controller\\Actuation Network\\PS-RA03B\\User-Defined Variables\\RRA03B-Reading"(w270) -> ()  [unwired: 1 in, 1 out]
                n176 = shared-variable "FOFB-Controller\\Actuation Network\\PS-RA03B\\User-Defined Variables\\ALV06A-Reading"(w269) -> ()  [unwired: 1 in, 1 out]
                n177 = shared-variable "FOFB-Controller\\Actuation Network\\PS-RA03B\\User-Defined Variables\\ALV06B-Reading"(w268) -> ()  [unwired: 1 in, 1 out]
                n178 = shared-variable "FOFB-Controller\\Actuation Network\\PS-RA03B\\User-Defined Variables\\ACH07A-Reading"(w267) -> ()  [unwired: 1 in, 1 out]
                n179 = shared-variable "FOFB-Controller\\Actuation Network\\PS-RA03B\\User-Defined Variables\\ACV07A-Reading"(w266) -> ()  [unwired: 1 in, 1 out]
                n180 = shared-variable "FOFB-Controller\\Actuation Network\\PS-RA03B\\User-Defined Variables\\ACH05B-Reading"(w265) -> ()  [unwired: 1 in, 1 out]
                n181 = shared-variable "FOFB-Controller\\Actuation Network\\PS-RA03B\\User-Defined Variables\\ACV05B-Reading"(w264) -> ()  [unwired: 1 in, 1 out]
                n182 = shared-variable "FOFB-Controller\\Actuation Network\\PS-RA03B\\User-Defined Variables\\PS-RA03B-Status"(w272) -> ()  [unwired: 1 in, 1 out]
              }
              frame condition #3 {
                n183 = shared-variable "FOFB-Controller\\Actuation Network\\PS-RA04B\\User-Defined Variables\\ACH08-Reading"(w280) -> ()  [unwired: 1 in, 1 out]
                n184 = shared-variable "FOFB-Controller\\Actuation Network\\PS-RA04B\\User-Defined Variables\\RRA04B-Reading"(w279) -> ()  [unwired: 1 in, 1 out]
                n185 = shared-variable "FOFB-Controller\\Actuation Network\\PS-RA04B\\User-Defined Variables\\ALV08A-Reading"(w278) -> ()  [unwired: 1 in, 1 out]
                n186 = shared-variable "FOFB-Controller\\Actuation Network\\PS-RA04B\\User-Defined Variables\\ALV08B-Reading"(w277) -> ()  [unwired: 1 in, 1 out]
                n187 = shared-variable "FOFB-Controller\\Actuation Network\\PS-RA04B\\User-Defined Variables\\ACH09A-Reading"(w276) -> ()  [unwired: 1 in, 1 out]
                n188 = shared-variable "FOFB-Controller\\Actuation Network\\PS-RA04B\\User-Defined Variables\\ACV09A-Reading"(w275) -> ()  [unwired: 1 in, 1 out]
                n189 = shared-variable "FOFB-Controller\\Actuation Network\\PS-RA04B\\User-Defined Variables\\ACH07B-Reading"(w274) -> ()  [unwired: 1 in, 1 out]
                n190 = shared-variable "FOFB-Controller\\Actuation Network\\PS-RA04B\\User-Defined Variables\\ACV07B-Reading"(w273) -> ()  [unwired: 1 in, 1 out]
                n191 = shared-variable "FOFB-Controller\\Actuation Network\\PS-RA04B\\User-Defined Variables\\PS-RA04B-Status"(w281) -> ()  [unwired: 1 in, 1 out]
              }
              frame condition #4 {
                n192 = shared-variable "FOFB-Controller\\Actuation Network\\PS-RA05B\\User-Defined Variables\\ACH10-Reading"(w289) -> ()  [unwired: 1 in, 1 out]
                n193 = shared-variable "FOFB-Controller\\Actuation Network\\PS-RA05B\\User-Defined Variables\\RRA05B-Reading"(w288) -> ()  [unwired: 1 in, 1 out]
                n194 = shared-variable "FOFB-Controller\\Actuation Network\\PS-RA05B\\User-Defined Variables\\ALV10A-Reading"(w287) -> ()  [unwired: 1 in, 1 out]
                n195 = shared-variable "FOFB-Controller\\Actuation Network\\PS-RA05B\\User-Defined Variables\\ALV10B-Reading"(w286) -> ()  [unwired: 1 in, 1 out]
                n196 = shared-variable "FOFB-Controller\\Actuation Network\\PS-RA05B\\User-Defined Variables\\ACH11A-Reading"(w285) -> ()  [unwired: 1 in, 1 out]
                n197 = shared-variable "FOFB-Controller\\Actuation Network\\PS-RA05B\\User-Defined Variables\\ACV11A-Reading"(w284) -> ()  [unwired: 1 in, 1 out]
                n198 = shared-variable "FOFB-Controller\\Actuation Network\\PS-RA05B\\User-Defined Variables\\ACH09B-Reading"(w283) -> ()  [unwired: 1 in, 1 out]
                n199 = shared-variable "FOFB-Controller\\Actuation Network\\PS-RA05B\\User-Defined Variables\\ACV09B-Reading"(w282) -> ()  [unwired: 1 in, 1 out]
                n200 = shared-variable "FOFB-Controller\\Actuation Network\\PS-RA05B\\User-Defined Variables\\PS-RA05B-Status"(w290) -> ()  [unwired: 1 in, 1 out]
              }
              frame condition #5 {
                n201 = shared-variable "FOFB-Controller\\Actuation Network\\PS-RA06B\\User-Defined Variables\\ACH12-Reading"(w298) -> ()  [unwired: 1 in, 1 out]
                n202 = shared-variable "FOFB-Controller\\Actuation Network\\PS-RA06B\\User-Defined Variables\\RRA06B-Reading"(w297) -> ()  [unwired: 1 in, 1 out]
                n203 = shared-variable "FOFB-Controller\\Actuation Network\\PS-RA06B\\User-Defined Variables\\ALV12A-Reading"(w296) -> ()  [unwired: 1 in, 1 out]
                n204 = shared-variable "FOFB-Controller\\Actuation Network\\PS-RA06B\\User-Defined Variables\\ALV12B-Reading"(w295) -> ()  [unwired: 1 in, 1 out]
                n205 = shared-variable "FOFB-Controller\\Actuation Network\\PS-RA06B\\User-Defined Variables\\ACH01A-Reading"(w294) -> ()  [unwired: 1 in, 1 out]
                n206 = shared-variable "FOFB-Controller\\Actuation Network\\PS-RA06B\\User-Defined Variables\\ACV01A-Reading"(w293) -> ()  [unwired: 1 in, 1 out]
                n207 = shared-variable "FOFB-Controller\\Actuation Network\\PS-RA06B\\User-Defined Variables\\ACH11B-Reading"(w292) -> ()  [unwired: 1 in, 1 out]
                n208 = shared-variable "FOFB-Controller\\Actuation Network\\PS-RA06B\\User-Defined Variables\\ACV11B-Reading"(w291) -> ()  [unwired: 1 in, 1 out]
                n209 = shared-variable "FOFB-Controller\\Actuation Network\\PS-RA06B\\User-Defined Variables\\PS-RA06B-Status"(w299) -> ()  [unwired: 1 in, 1 out]
              }
            }
          }
        }
      }
    }
  }
